vi "Configure Trigger Source.vi"(8 "error in (no error)":errorcluster, 9 "Internal Trigger Source (1: Pulse Sync)":i32(ring)=1 items=["Pulse Video", "Pulse Sync"], 10 "External Trigger Source (0: Trigger1)":i32(ring) items=["Trigger1", "Trigger2", "Pulse"], 11 "VISA resource name":refnum<visa-resource-name>) -> (0 "error out":errorcluster, 3 "VISA resource name out":refnum<visa-resource-name>)   [LabVIEW 2012, in "Agilent PSG MXG Series.lvlib"]
doc: "Selects the external/internal trigger source.\n\n<B>Notes:</B>\n(1) This VI is valid only in N5162A, N5182A, N5172B, N5182B."
uses:
  <instrlib>/Agilent PSG MXG Series/Agilent PSG MXG Series.lvlib
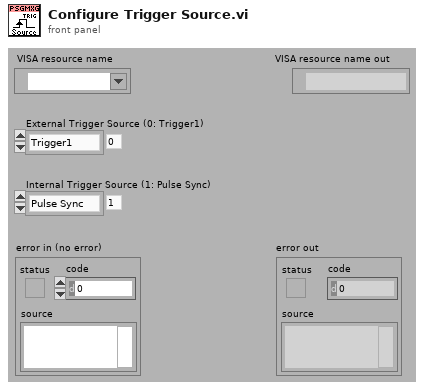
[diagram p1: front panel]
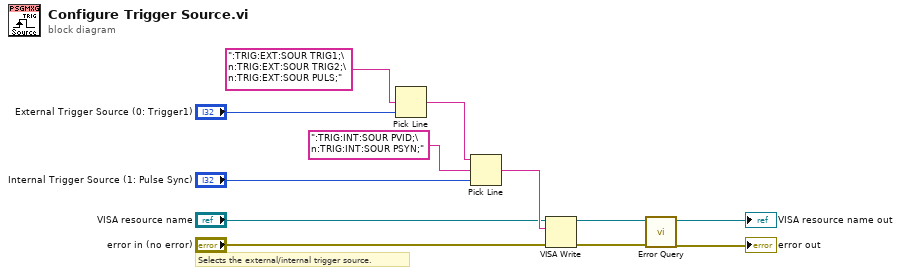
[diagram p0: block diagram]
diagram:
  # "Selects the external/internal trigger source."
  n1 = Pick Line(multi-line string=":TRIG:EXT:SOUR TRIG1;\n:TRIG:EXT:SOUR TRIG2;\n:TRIG:EXT:SOUR PULS;", line index="External Trigger Source (0: Trigger1)") -> (output string=w8:string)  [unwired: 1 out]
  n2 = Pick Line(string ("")=w8, multi-line string=":TRIG:INT:SOUR PVID;\n:TRIG:INT:SOUR PSYN;", line index="Internal Trigger Source (1: Pulse Sync)") -> (output string=w7:string)
  n3 = VISA Write(VISA resource name="VISA resource name", write buffer=w7, error in (no error)="error in (no error)") -> (VISA resource name out=w4:refnum<visa-resource-name>, error out=w3:errorcluster)  [unwired: 1 out]
  n4 = call <instrlib>:"Error Query.vi"("error in (no error)"=w3, "VISA resource name"=w4) -> ("error out"=→"error out":errorcluster, "VISA resource name out"=→"VISA resource name out":refnum<visa-resource-name>)  [unwired: 8 out]
